vi "Update main window size.vi"(8 "error in (no error)":errorcluster, 11 "DAQOrcaFlash in":refnum<class "DAQOrcaFlash.lvclass">) -> (0 "error out":errorcluster, 3 "DAQOrcaFlash out":refnum<class "DAQOrcaFlash.lvclass">)   [LabVIEW 2012, in "DAQOrcaFlash.lvclass"]
uses:
  DAQOrcaFlash.lvclass
  DAQOrcaFlash.lvclass/DAQOrcaFlash.ctl
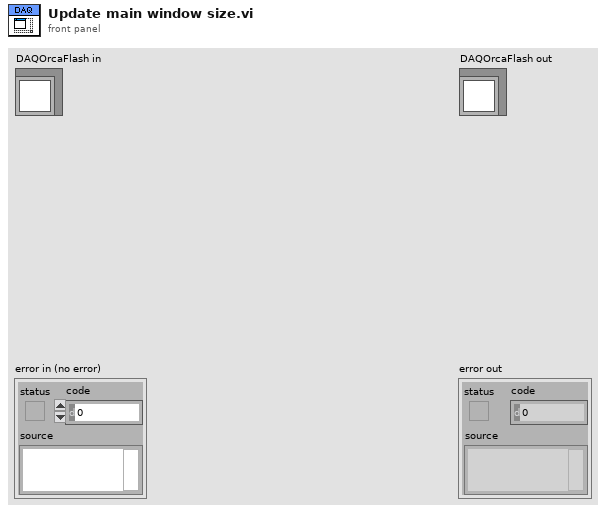
[diagram p1: front panel]
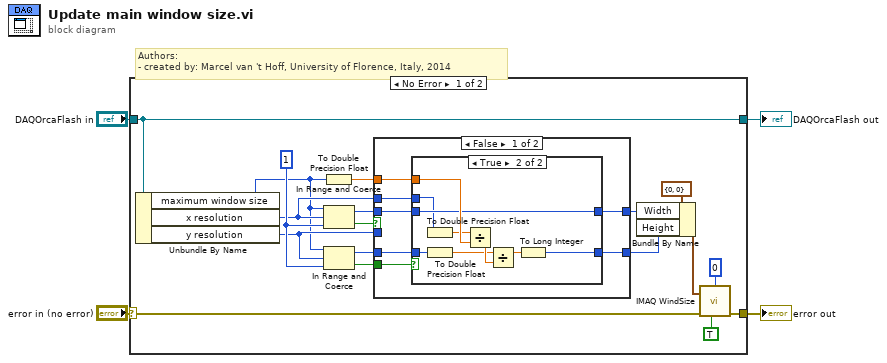
[diagram p0: block diagram]
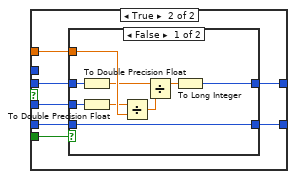
[diagram p3: hidden frame]
diagram:
  # "Authors: \n- created by: Marcel van 't Hoff, University of Florence, Italy, 2014"
  n1 = case shown="No Error" "error in (no error)" {
    selector: "error in (no error)" -> [w17 w60]
    tunnel: [w16 w60] -> w3
    tunnel: [w22 w59] -> w1
    tunnel: "DAQOrcaFlash in" -> [w22 w59]
    frame No Error {
      w21 = 1 ("lower limit")
      n2 = Unbundle By Name(w22) -> ("maximum window size"=w5:i32, "x resolution"=w7:i32, "y resolution"=w6:i32)
      n3 = To Double Precision Float(number=w5) -> (double precision float=w10:dbl)
      n4 = In Range and Coerce(upper limit=w5, x=w7, lower limit=w21) -> (coerced(x)=w13:i32, In Range?=w14:bool)
      n5 = In Range and Coerce(upper limit=w5, x=w6, lower limit=w21) -> (coerced(x)=w12:i32, In Range?=w11:bool)
      n6 = case shown="False" w14 {
        tunnel: w13 -> [w27 w45]
        tunnel: w12 -> [w25 w43]
        tunnel: w11 -> [w29 w47]
        tunnel: [w28 w46] -> w9
        tunnel: [w26 w44] -> w8
        tunnel: w10 -> [w24 w42]
        tunnel: w7 -> [w23 _]
        tunnel: w6 -> [_ w41]
        frame False {
          n7 = case shown="True" w29 {
            tunnel: [w31 w33] -> w28
            tunnel: w27 -> [w31 w33]
            tunnel: [w30 w34] -> w26
            tunnel: w25 -> [w30 w37]
            tunnel: w24 -> [_ w40]
            tunnel: w23 -> [_ w32]
            frame False {
            }
            frame True {
              n8 = To Double Precision Float(number=w32) -> (double precision float=w38:dbl)
              n9 = To Double Precision Float(number=w37) -> (double precision float=w36:dbl)
              n10 = Divide(x=w38, y=w40) -> (x/y=w39:dbl)
              n11 = Divide(x=w36, y=w39) -> (x/y=w35:dbl)
              n12 = To Long Integer(number=w35) -> (32bit integer=w34:i32)
            }
          }
        }
        frame True {
          n13 = case shown="False" w47 {
            tunnel: [w50 w58] -> w46
            tunnel: w45 -> [w51 w58]
            tunnel: [w49 w57] -> w44
            tunnel: w43 -> [w49 w57]
            tunnel: w42 -> [w56 _]
            tunnel: w41 -> [w48 _]
            frame False {
              n14 = To Double Precision Float(number=w51) -> (double precision float=w53:dbl)
              n15 = To Double Precision Float(number=w48) -> (double precision float=w54:dbl)
              n16 = Divide(x=w54, y=w56) -> (x/y=w55:dbl)
              n17 = Divide(x=w53, y=w55) -> (x/y=w52:dbl)
              n18 = To Long Integer(number=w52) -> (32bit integer=w50:i32)
            }
            frame True {
            }
          }
        }
      }
      n19 = Bundle By Name(cluster=cluster{"Width":i32, "Height":i32} {"Width"=0, "Height"=0} ("Width & Height"), "Width"=w9, "Height"=w8) -> (w19:cluster{"Width":i32, "Height":i32})
      n20 = call "IMAQ WindSize"("error in (no error)"=w17, "Get/Set Status? (Set)"=TRUE, "Width & Height"=w19, "Window Number"=0) -> ("error out"=w16:errorcluster)  [unwired: 2 in, 2 out]
    }
    frame Error {
    }
  }
  "error out" <- w3
  "DAQOrcaFlash out" <- w1
